vi "Auto Zoom Query.vi"(8 "error in":errorcluster, 11 "Instrument Handle In":i32) -> (0 "error out":errorcluster, 1 "Stop":dbl, 2 "Start":dbl, 3 "Instrument Handle Out":i32)   [LabVIEW 8.6, in "ZTScopeM.lvlib"]
doc: "Query the auto download buffer zoom level. A start and stop that are equal to the capture time (0 to sweep time) will cause a single waveform to be available in the auto download buffer. A different start and stop time will provide a secondary \"zoomed\" waveform within the selected times."
uses:
  ZTScopeM.lvlib
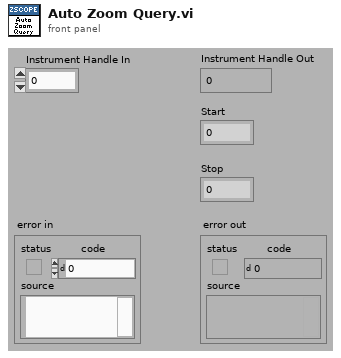
[diagram p1: front panel]
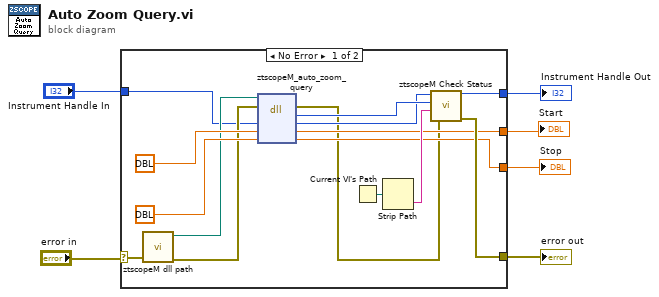
[diagram p0: block diagram]
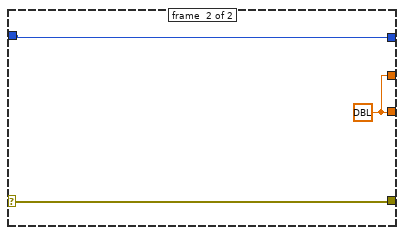
[diagram p2: hidden frame]
diagram:
  n1 = case shown="No Error" "error in" {
    selector: "error in" -> [w11 w24]
    tunnel: [w16 w24] -> w5
    tunnel: [w17 w22] -> w4
    tunnel: [w14 w23] -> w3
    tunnel: [w12 w23] -> w2
    tunnel: "Instrument Handle In" -> [w7 w22]
    frame #0 {
      n2 = call "ztscopeM dll path.vi"("error in (no error)"=w11) -> ("error out"=w9:errorcluster, "<instrument>.dll path"=w10:path)  [unwired: 9 in]
      n3 = dll-call lib="C:/Program Files (x86)/National Instruments/LabVIEW 2013/instr.lib/ztscopem/ztscopeM.dll" fn="ztscopeM_auto_zoom_query"(path in=w10, error in=w9, "instrumentHandle"=w7, "Start"=dbl ? ("Start in"), "Stop"=dbl ? ("Stop in")) -> (error out=w8:errorcluster, "return type"=w21:i32, "instrumentHandle"=w20:i32, "Start"=w12:dbl, "Stop"=w14:dbl)  [unwired: 1 in, 1 out]
      n4 = Current VI's Path() -> (path=w19:path)
      n5 = Strip Path(path=w19) -> (name=w18:string)  [unwired: 1 out]
      n6 = call "ztscopeM Check Status.vi"("error in"=w8, "name of VI"=w18, "status (return code)"=w21, "instrument handle in"=w20) -> ("error out"=w16:errorcluster, "instrument handle out"=w17:i32)  [unwired: 2 out]
    }
    frame #1 {
      w23 = dbl ? ("Stop")
    }
  }
  "Instrument Handle Out" <- w4
  "error out" <- w5
  "Stop" <- w3
  "Start" <- w2
